vi "Read Custom Errors.vi"(8 "error in (no error)":errorcluster, 11 "Custom Errors in":refnum<class "Custom Errors.lvclass">) -> (0 "error out":errorcluster, 2 "Custom Errors":T1[](array[typedef]), 3 "Custom Errors out":refnum<class "Custom Errors.lvclass">)   [LabVIEW 2021, in "TAF Proj Document Type.lvlib" / "Custom Errors.lvclass"]
uses:
  <vilib>/Wovalab/AntiDoc/Document Type/Add-ons/LabVIEW TAF Project/Custom Errors/Custom Errors.lvclass
  <vilib>/Wovalab/AntiDoc/Bloc/Custom Error Info--cluster.ctl
  <vilib>/Wovalab/AntiDoc/Document Type/Add-ons/LabVIEW TAF Project/Custom Errors/Custom Errors.lvclass/Custom Errors.ctl
  <vilib>/Wovalab/AntiDoc/Bloc/Bloc.lvclass
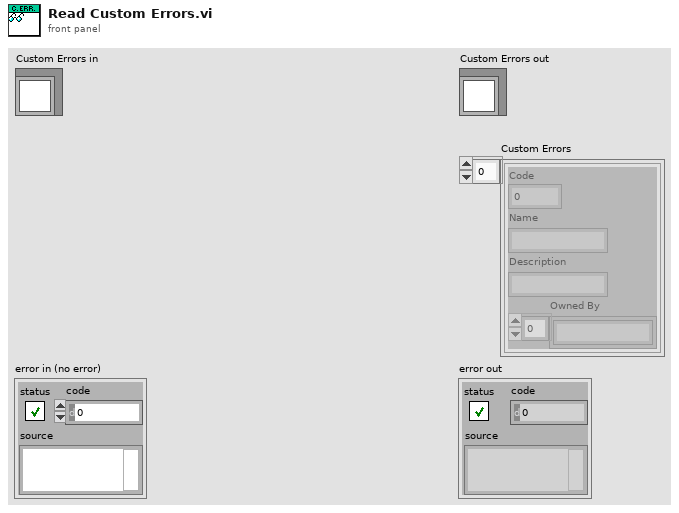
[diagram p1: front panel]
types:
  T1 = typedef "AntiDoc.lvlib/Bloc.lvclass/Custom Error Info--cluster.ctl" = cluster{"Code":i32, "Name":string, "Description":string, "Owned By":string[]}
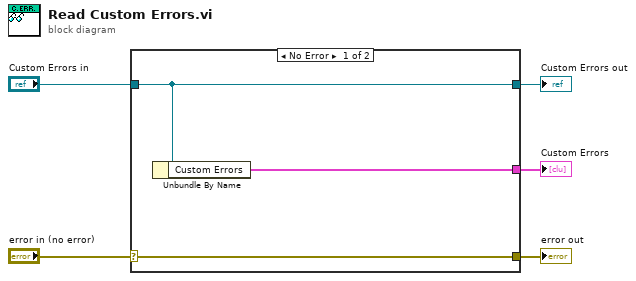
[diagram p0: block diagram]
diagram:
  n1 = case shown="No Error" "error in (no error)" {
    selector: "error in (no error)" -> [w8 w9]
    tunnel: [w8 w9] -> w4
    tunnel: [w7 w10] -> w2
    tunnel: "Custom Errors in" -> [w7 w10]
    tunnel: [w6 _] -> w1
    frame No Error {
      n2 = Unbundle By Name(w7) -> ("Custom Errors"=w6:T1[])
    }
    frame Error {
    }
  }
  "error out" <- w4
  "Custom Errors out" <- w2
  "Custom Errors" <- w1
